vi "sub_prepare_outputfiles.vi"(8 "error in":errorcluster, 10 "Dynamic data in":T1, 11 "Input parameters 2":T2={"Measurement type"=enum."Debug", "Sensor type"=enum."HPK_8in_256", "Identifier"="test.txt", "Open after execution?"=FALSE, "Plot after execution?"=FALSE, "Display channel"=0, "Voltage Delay (s)"=0.5, "Switch Delay (s)"=0.01, "VISA resource name source"="", "VISA resource name DMM"="", "VISA resource name LCR"="", "Compliance  Level (A)"=10.0, "Voltage Limit (V)"=1000.0, "Data storage location"="", "Scan voltages"="", "Use source as DMM?"=FALSE, "LCR signal frequenzy (Hz)"=10.0, "DMM device"=enum."Keithley2001", "Sampling number"=1, "Use env. sensors on"=enum."Sensirion sht1x/7x", "Switchboard Handle"=0, "Use Switchboard"=FALSE, "LCR signal voltage (V)"=10000.0, "Repeat"=1, "Scan voltages IV"="", "Scan voltages CV"="", "Hex pad numbers?"=FALSE, "Set measurement type"=enum."Debug", "Custom pad scan"="", "IV voltage Delay (s)"=0.5, "CV voltage Delay (s)"=0.5, "Needle measurement?"=FALSE, "Comments"="test.txt", "LCR signal frequenzy (kHz)"=10.0, "Compliance  Level (uA)"=10.0, "Open Correction Array"=array2304x3[6912 elements], "Current set voltage"=0.0, "Last set voltage"=0.0, "Current channel"=0, "Last OpenCorrection index"=-1, "Total curr/vltg every x steps"=10, "Current channel iteration"=0, "No CV corrections"=FALSE, "Mapfile"="", "Corrfile"="", "IV voltage file"=path "", "CV voltage file"=path "", "IV Switch Delay (s)"=0.01, "CV Switch Delay (s)"=0.01} {"CV Switch Delay (s)" format="%#_13g"; "IV Switch Delay (s)" format="%#_13g"; "Last set voltage" format="%#_13g"; "Current set voltage" format="%#_13g"; "CV voltage Delay (s)" format="%#_13g"; "IV voltage Delay (s)" format="%#_13g"; "Voltage Limit (V)" format="%#_13g"; "Voltage Delay (s)" format="%#_13g"; "Switch Delay (s)" format="%#_13g"}) -> (0 "error out":errorcluster, 2 "Dynamic data out":T1, 3 "Input parameters":T2={"Measurement type"=enum."Debug", "Sensor type"=enum."HPK_8in_256", "Identifier"="test.txt", "Open after execution?"=FALSE, "Plot after execution?"=FALSE, "Display channel"=0, "Voltage Delay (s)"=0.5, "Switch Delay (s)"=0.01, "VISA resource name source"="", "VISA resource name DMM"="", "VISA resource name LCR"="", "Compliance  Level (A)"=10.0, "Voltage Limit (V)"=1000.0, "Data storage location"="", "Scan voltages"="", "Use source as DMM?"=FALSE, "LCR signal frequenzy (Hz)"=10.0, "DMM device"=enum."Keithley2001", "Sampling number"=1, "Use env. sensors on"=enum."Sensirion sht1x/7x", "Switchboard Handle"=0, "Use Switchboard"=FALSE, "LCR signal voltage (V)"=10000.0, "Repeat"=1, "Scan voltages IV"="", "Scan voltages CV"="", "Hex pad numbers?"=FALSE, "Set measurement type"=enum."Debug", "Custom pad scan"="", "IV voltage Delay (s)"=0.5, "CV voltage Delay (s)"=0.5, "Needle measurement?"=FALSE, "Comments"="test.txt", "LCR signal frequenzy (kHz)"=10.0, "Compliance  Level (uA)"=10.0, "Open Correction Array"=array2304x3[6912 elements], "Current set voltage"=0.0, "Last set voltage"=0.0, "Current channel"=0, "Last OpenCorrection index"=-1, "Total curr/vltg every x steps"=10, "Current channel iteration"=0, "No CV corrections"=FALSE, "Mapfile"="", "Corrfile"="", "IV voltage file"=path "", "CV voltage file"=path "", "IV Switch Delay (s)"=0.01, "CV Switch Delay (s)"=0.01} {"CV Switch Delay (s)" format="%#_13g"; "IV Switch Delay (s)" format="%#_13g"; "Last set voltage" format="%#_13g"; "Current set voltage" format="%#_13g"; "CV voltage Delay (s)" format="%#_13g"; "IV voltage Delay (s)" format="%#_13g"; "Voltage Limit (V)" format="%#_13g"; "Voltage Delay (s)" format="%#_13g"; "Switch Delay (s)" format="%#_13g"})   [LabVIEW 2016]
uses:
  input_params.ctl
  data_dynamic.ctl
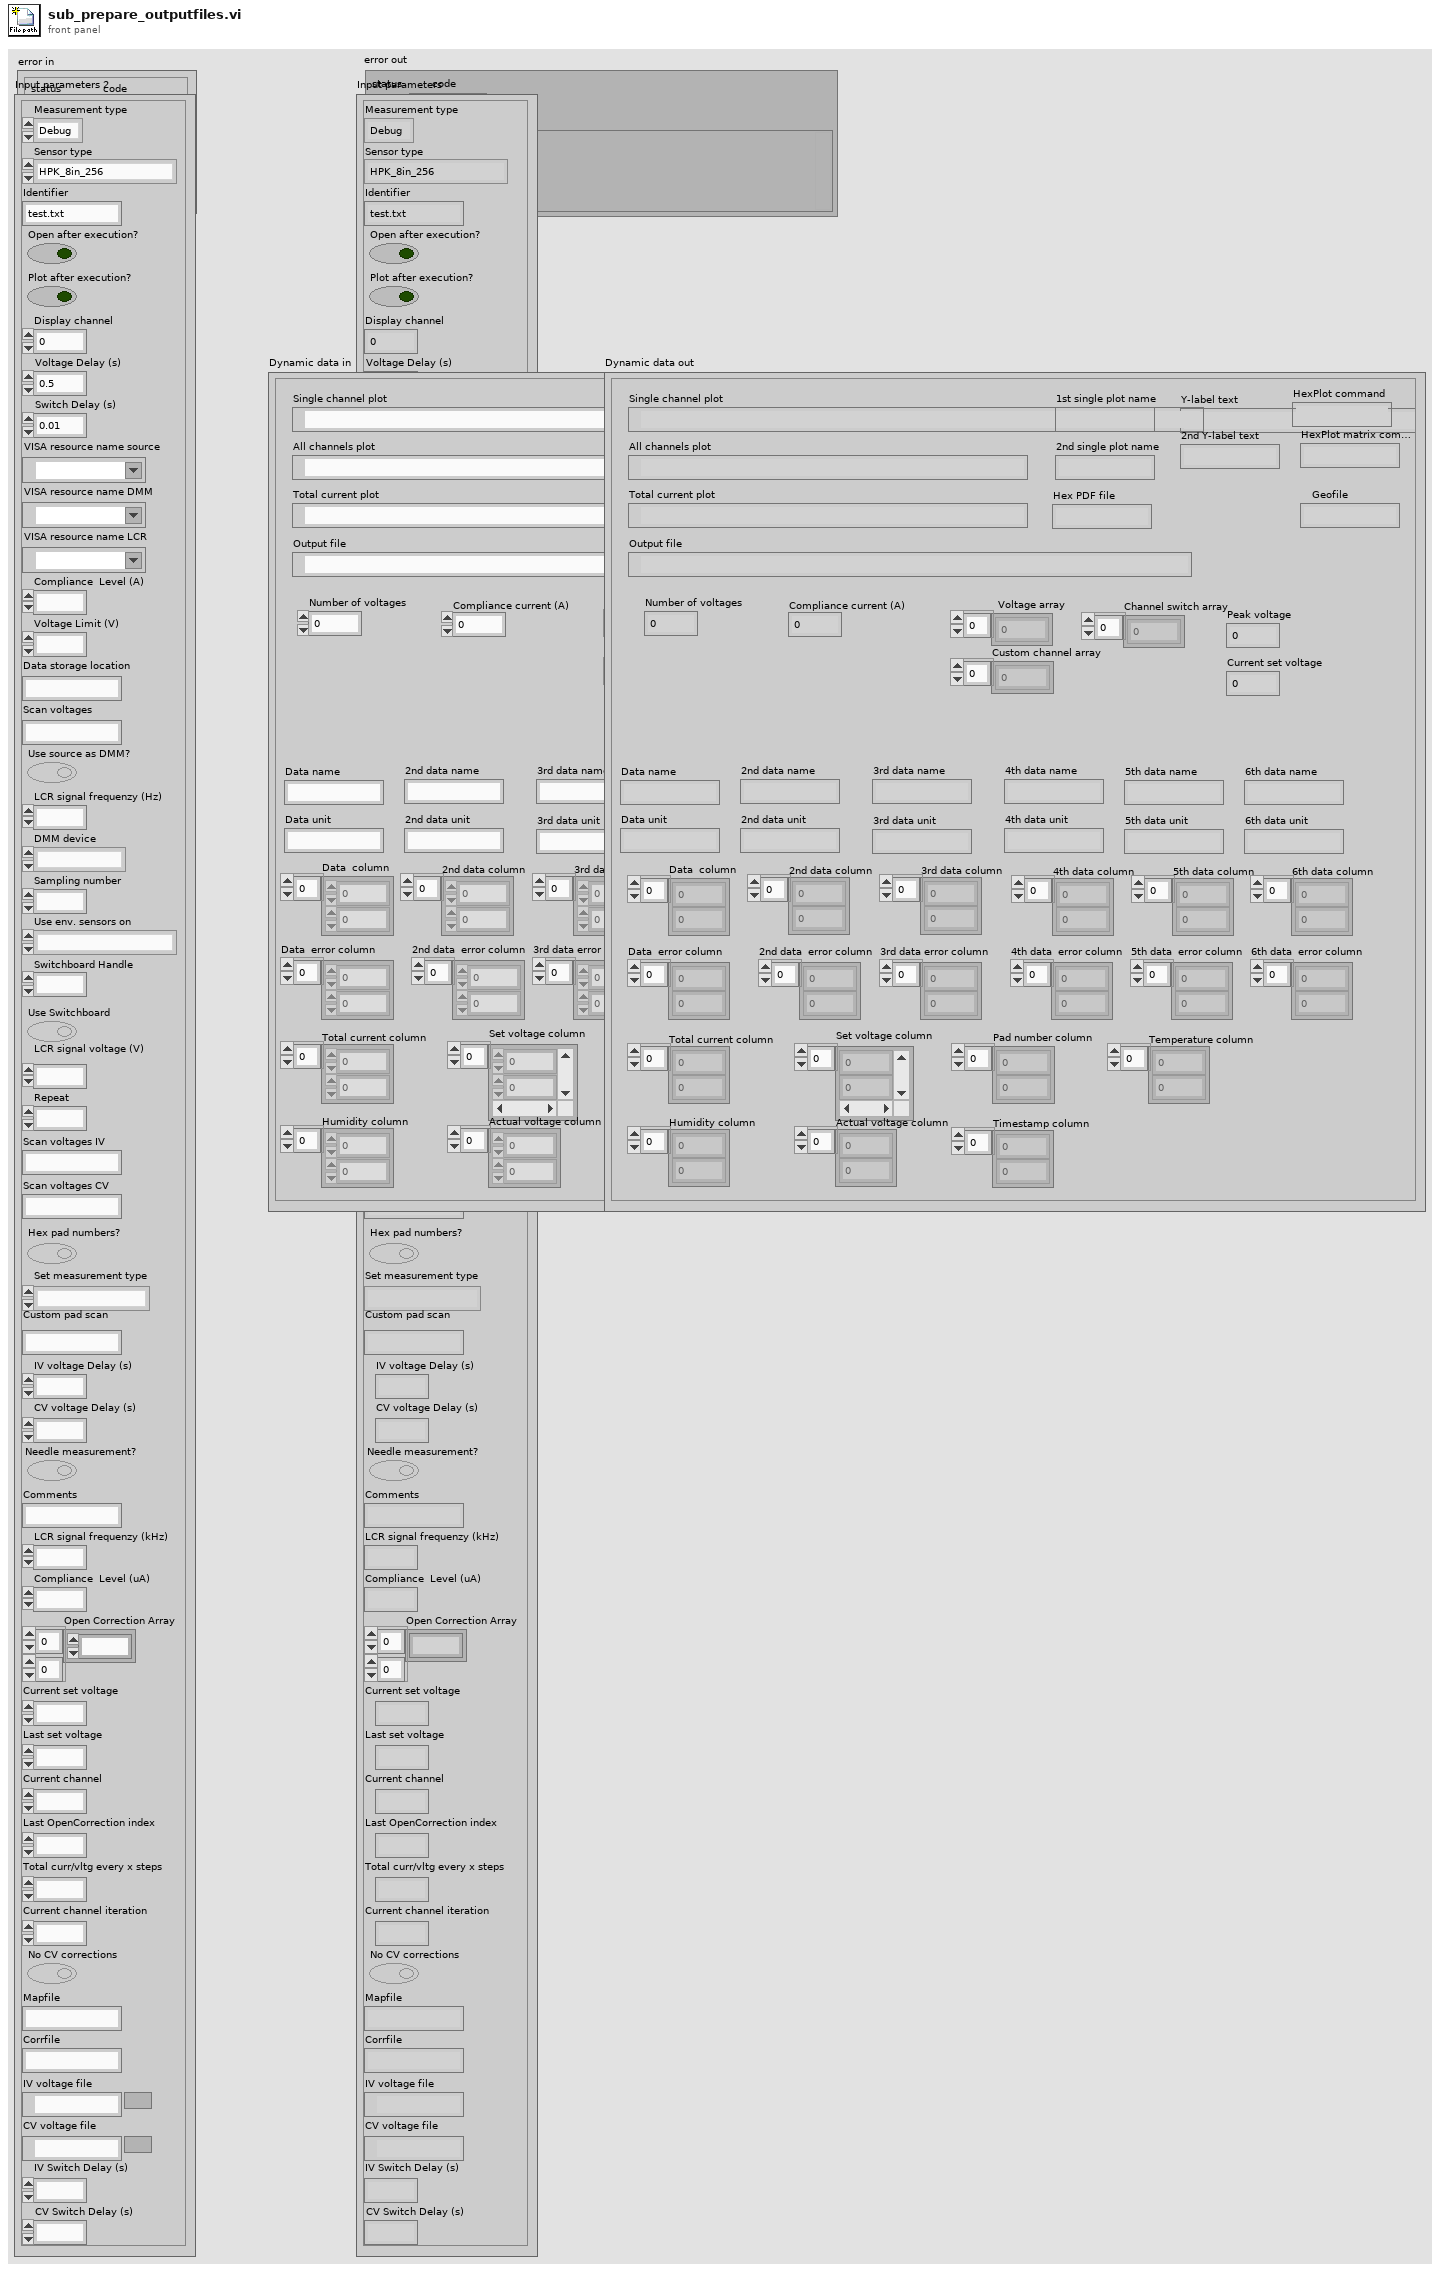
[diagram p1: front panel]
types:
  T1 = typedef "data_dynamic.ctl" = cluster{"Output file":path, "Y-label text":string, "Current set voltage":dbl, "Set voltage column":dbl[], "Pad number column":dbl[], "Data  column":dbl[], "Number of voltages":i32, "Compliance current (A)":dbl, "Geofile":string, "Peak voltage":dbl, "Hex PDF file":string, "Voltage array":dbl[], "Total current column":dbl[], "Timestamp column":dbl[], "Data name":string, "Data unit":string, "2nd data column":dbl[], "2nd data name":string, "2nd data unit":string, "3rd data column":dbl[], "4th data column":dbl[], "3rd data name":string, "3rd data unit":string, "4th data name":string, "4th data unit":string, "Actual voltage column":dbl[], "2nd Y-label text":string, "Single channel plot":path, "Temperature column":dbl[], "Humidity column":dbl[], "Channel switch array":i32[], "1st single plot name":string, "2nd single plot name":string, "All channels plot":path, "HexPlot command":string, "Custom channel array":i32[], "Data  error column":dbl[], "2nd data  error column":dbl[], "3rd data error column":dbl[], "4th data  error column":dbl[], "Total current plot":path, "5th data column":dbl[], "5th data  error column":dbl[], "6th data column":dbl[], "6th data  error column":dbl[], "5th data name":string, "5th data unit":string, "6th data name":string, "6th data unit":string, "HexPlot matrix command":string}
  T2 = typedef "input_params.ctl" = cluster{"Measurement type":enum16{"IV", "CV", "Debug", "Test_contact"}, "Sensor type":enum16{"HPK_6in_135", "HPK_8in_256", "IFX_8in_256", "Diode", "HPK_6in_256", "Full matrix"}, "Identifier":string, "Open after execution?":bool, "Plot after execution?":bool, "Display channel":i32, "Voltage Delay (s)":dbl, "Switch Delay (s)":dbl, "VISA resource name source":refnum<visa-resource-name>, "VISA resource name DMM":refnum<visa-resource-name>, "VISA resource name LCR":refnum<visa-resource-name>, "Compliance  Level (A)":dbl, "Voltage Limit (V)":dbl, "Data storage location":string, "Scan voltages":string, "Use source as DMM?":bool, "LCR signal frequenzy (Hz)":dbl, "DMM device":enum16{"Keithley2001", "Keithley2450", "Keithley2410", "Keithley6487"}, "Sampling number":i32, "Use env. sensors on":enum16{"Sensirion sht1x/7x", "Switch Matrix", "Probecard"}, "Switchboard Handle":u32, "Use Switchboard":bool, "LCR signal voltage (V)":dbl, "Repeat":i32, "Scan voltages IV":string, "Scan voltages CV":string, "Hex pad numbers?":bool, "Set measurement type":enum16{"IV", "CV", "Debug", "Test_contact", "IV+CV"}, "Custom pad scan":string, "IV voltage Delay (s)":dbl, "CV voltage Delay (s)":dbl, "Needle measurement?":bool, "Comments":string, "LCR signal frequenzy (kHz)":dbl, "Compliance  Level (uA)":dbl, "Open Correction Array":dbl[][], "Current set voltage":dbl, "Last set voltage":dbl, "Current channel":i32, "Last OpenCorrection index":i32, "Total curr/vltg every x steps":i32, "Current channel iteration":i32, "No CV corrections":bool, "Mapfile":string, "Corrfile":string, "IV voltage file":path, "CV voltage file":path, "IV Switch Delay (s)":dbl, "CV Switch Delay (s)":dbl}
  T3 = enum16{"IV", "CV", "Debug", "Test_contact", "IV+CV"}
  T4 = enum16{"HPK_6in_135", "HPK_8in_256", "IFX_8in_256", "Diode", "HPK_6in_256", "Full matrix"}
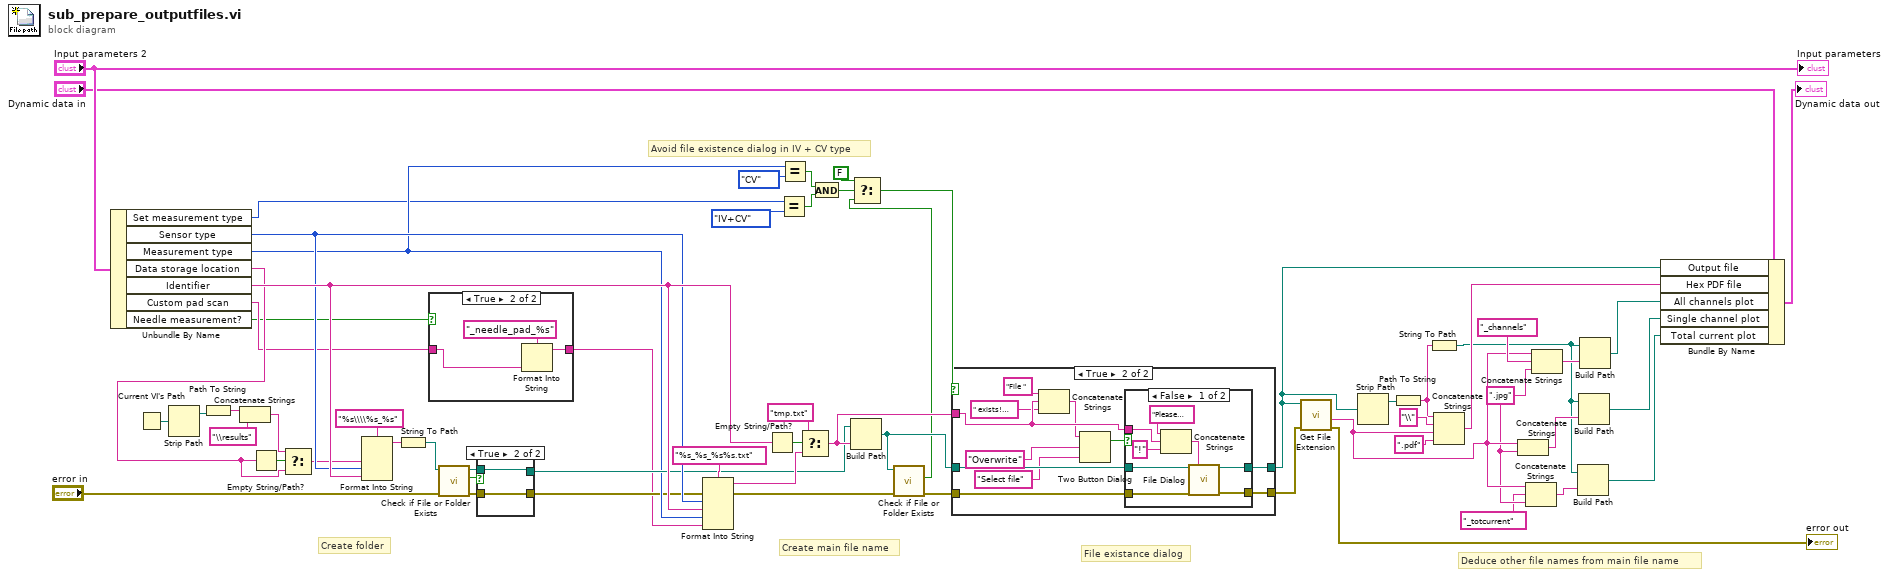
[diagram p0: block diagram]
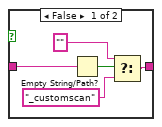
[diagram p2: hidden frame]
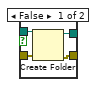
[diagram p3: hidden frame]
diagram:
  w4 = ".jpg" ("string")
  # "Deduce other file names from main file name"
  # "File existance dialog"
  # "Create main file name"
  # "Create folder"
  # "Avoid file existence dialog in IV + CV type"
  n1 = Unbundle By Name("Input parameters 2") -> ("Set measurement type"=w15:T3, "Sensor type"=w35:T4, "Measurement type"=w27:enum16{"IV", "CV", "Debug", "Test_contact"}, "Data storage location"=w11:string, "Identifier"=w36:string, "Custom pad scan"=w9:string, "Needle measurement?"=w1:bool)
  n2 = Current VI's Path() -> (path=w58:path)
  n3 = Strip Path(path=w58) -> (stripped path=w57:path)  [unwired: 1 out]
  n4 = Path To String(path=w57) -> (string=w56:string)
  n5 = Concatenate Strings(w56, "\\results" ("string")) -> (w54:string)
  n6 = Empty String/Path?(string/path=w11) -> (empty?=w59:bool)
  n7 = Select(t=w54, s=w59, f=w11) -> (s? t:f=w34:string)
  n8 = Format Into String(format string="%s\\\\%s_%s", w34, w35, w36) -> (resulting string=w33:string)  [unwired: 2 in, 1 out]
  n9 = String To Path(string=w33) -> (path=w31:path)
  n10 = case shown="True" w1 {
    tunnel: w9 -> [w67 w70]
    tunnel: [w63 w69] -> w8
    frame False {
      n11 = Empty String/Path?(string/path=w67) -> (empty?=w66:bool)
      n12 = Select(t="" ("format string"), s=w66, f="_customscan" ("format string")) -> (s? t:f=w63:string)
    }
    frame True {
      n13 = Format Into String(format string="_needle_pad_%s", w70) -> (resulting string=w69:string)  [unwired: 2 in, 1 out]
    }
  }
  n14 = call <vilib>:"Check if File or Folder Exists.vi"("error in (no error)"="error in", "path"=w31) -> ("error out"=w14:errorcluster, "file or folder exists?"=w30:bool, "dup path"=w29:path)  [unwired: 7 in]
  n15 = case shown="True" w30 {
    tunnel: w29 -> [w74 w76]
    tunnel: [w73 w76] -> w28
    tunnel: w14 -> [w72 w75]
    tunnel: [w71 w75] -> w12
    frame False {
      n16 = Create Folder(path (use dialog)=w74, error in=w72) -> (created path=w73:path, error out=w71:errorcluster)  [unwired: 1 in, 1 out]
    }
    frame True {
    }
  }
  n17 = Format Into String(format string="%s_%s_%s%s.txt", error in=w12, w35, w36, w27, w8) -> (resulting string=w50:string, error out=w37:errorcluster)  [unwired: 1 in]
  n18 = Empty String/Path?(string/path=w36) -> (empty?=w53:bool)
  n19 = Equal?(x=w15, y=enum16{"IV", "CV", "Debug", "Test", "IV+CV"}."IV+CV") -> (x = y?=w23:bool)
  n20 = Equal?(x=w27, y=enum16{"IV", "CV", "Debug", "Test"}."CV") -> (x = y?=w22:bool)
  n21 = Select(t="tmp.txt", s=w53, f=w50) -> (s? t:f=w47:string)
  n22 = And(x=w22, y=w23) -> (x .and. y?=w24:bool)
  n23 = Build Path(base path=w28, name or relative path=w47) -> (appended path=w49:path)
  n24 = call <vilib>:"Check if File or Folder Exists.vi"("error in (no error)"=w37, "path"=w49) -> ("error out"=w48:errorcluster, "file or folder exists?"=w20:bool)  [unwired: 7 in, 1 out]
  n25 = Select(t=FALSE, s=w24, f=w20) -> (s? t:f=w19:bool)
  n26 = case shown="True" w19 {
    tunnel: w49 -> [w78 w89]
    tunnel: [w78 w88] -> w46
    tunnel: w48 -> [w77 w87]
    tunnel: [w77 w86] -> w42
    tunnel: w47 -> [_ w85]
    frame False {
    }
    frame True {
      n27 = Concatenate Strings("File " ("string"), w85, " exists! Overwite?" ("string")) -> (w82:string)
      n28 = Two Button Dialog(message=w82, 1:"Select file" ("Center Button Text (\"No\")"), 2:"Overwrite" ("Left Button Text (\"Yes\")")) -> (T button?=w79:bool)
      n29 = case shown="False" w79 {
        tunnel: w89 -> [w97 w99]
        tunnel: [w96 w99] -> w88
        tunnel: w87 -> [w95 w98]
        tunnel: [w94 w98] -> w86
        tunnel: w85 -> [w91 _]
        frame False {
          n30 = Concatenate Strings("Please chose a new file instead of  " ("prompt (Choose or enter file path)"), w91, "!" ("string")) -> (w93:string)
          n31 = call "File Dialog"("start path"=w97, "prompt"=w93, "error in"=w95) -> ("selected path"=w96:path, "error out"=w94:errorcluster)  [unwired: 9 in, 2 out]
        }
        frame True {
        }
      }
    }
  }
  n32 = call <vilib>:"Get File Extension.vi"("error in (no error)"=w42, "file"=w46) -> ("error out"=→"error out":errorcluster, "filename without extension"=w5:string)  [unwired: 5 in, 3 out]
  n33 = Strip Path(path=w46) -> (stripped path=w61:path)  [unwired: 1 out]
  n34 = Path To String(path=w61) -> (string=w43:string)
  n35 = String To Path(string=w43) -> (path=w7:path)
  n36 = Concatenate Strings(w43, "\\" ("string"), w5, ".pdf" ("string")) -> (w45:string)
  n37 = Concatenate Strings(w5, w4) -> (w44:string)
  n38 = Concatenate Strings(w5, "_totcurrent" ("string"), w4) -> (w6:string)
  n39 = Concatenate Strings(w5, "_channels" ("string"), w4) -> (w41:string)
  n40 = Build Path(base path=w7, name or relative path=w6) -> (appended path=w2:path)
  n41 = Build Path(base path=w7, name or relative path=w44) -> (appended path=w39:path)
  n42 = Build Path(base path=w7, name or relative path=w41) -> (appended path=w38:path)
  n43 = Bundle By Name(cluster="Dynamic data in", "Output file"=w46, "Hex PDF file"=w45, "All channels plot"=w38, "Single channel plot"=w39, "Total current plot"=w2) -> (→"Dynamic data out":T1)
  "Input parameters" <- "Input parameters 2"
